vi "Diff Tree Items.vi"(10 "New Items":T1(array[cluster])=[{"Parent Tag"="", "Child Tag"="C:\\Users\\zwatx\\Developer\\LabView\\2026\\rebuilt-2687\\Robot Code\\Paths\\Choreo", "Left Cell Text"="Choreo", "Column Texts[]"=[], "Is File"=FALSE}, {"Parent Tag"="C:\\Users\\zwatx\\Developer\\LabView\\2026\\rebuilt-2687\\Robot Code\\Paths\\Choreo", "Child Tag"="C:\\Users\\zwatx\\Developer\\LabView\\2026\\rebuilt-2687\\Robot Code\\Paths\\Choreo\\Test", "Left Cell Text"="Test", "Column Texts[]"=[], "Is File"=FALSE}, {"Parent Tag"="", "Child Tag"="C:\\Users\\zwatx\\Developer\\LabView\\2026\\rebuilt-2687\\Robot Code\\Paths\\Hi", "Left Cell Text"="Hi", "Column Texts[]"=[], "Is File"=FALSE}], 11 "Old Items":T1(array[cluster])=[{"Parent Tag"="", "Child Tag"="C:\\Users\\zwatx\\Developer\\LabView\\2026\\rebuilt-2687\\Robot Code\\Paths\\Choreo", "Left Cell Text"="Choreo", "Column Texts[]"=[], "Is File"=FALSE}, {"Parent Tag"="C:\\Users\\zwatx\\Developer\\LabView\\2026\\rebuilt-2687\\Robot Code\\Paths\\Choreo", "Child Tag"="C:\\Users\\zwatx\\Developer\\LabView\\2026\\rebuilt-2687\\Robot Code\\Paths\\Choreo\\Test", "Left Cell Text"="Test", "Column Texts[]"=[], "Is File"=FALSE}, {"Parent Tag"="", "Child Tag"="C:\\Users\\zwatx\\Developer\\LabView\\2026\\rebuilt-2687\\Robot Code\\Paths\\Hi", "Left Cell Text"="Hi", "Column Texts[]"=[], "Is File"=FALSE}]) -> (1 "Removed Items":T1(array[cluster]), 2 "Changed Items":T1(array[cluster]), 3 "Added Items":T1(array[cluster]))   [LabVIEW 2025]
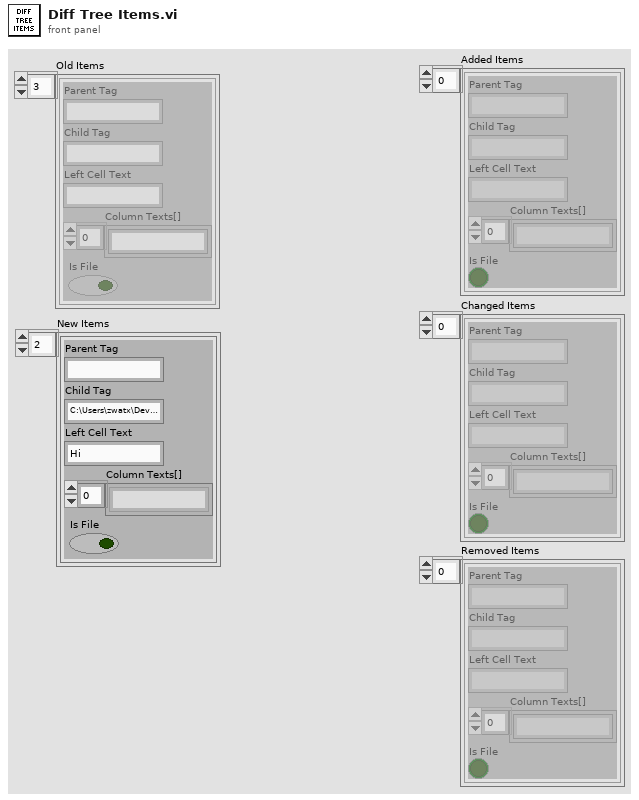
[diagram p1: front panel]
types:
  T1 = cluster{"Parent Tag":string, "Child Tag":string, "Left Cell Text":string, "Column Texts[]":string[], "Is File":bool}[]
  T2 = cluster{"Parent Tag":string, "Child Tag":string, "Left Cell Text":string, "Column Texts[]":string[], "Is File":bool}
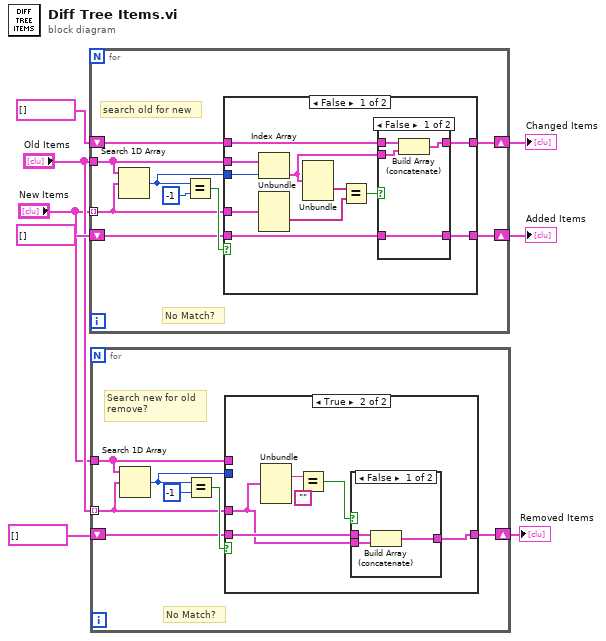
[diagram p0: block diagram]
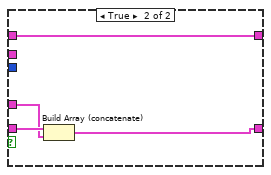
[diagram p5: hidden frame]
diagram:
  n1 = for {
    tunnel: "New Items" -> [w14] mode=indexing
    tunnel: "Old Items" -> [w12]
    shift-right: [w13] -> w7
    shift-left: T1 [] ("Old Items") -> [w15]
    shift-right: [w9] -> w5
    shift-left: T1 [] ("Old Items") -> [w10]
    # "search old for new"
    # "No Match?"
    n2 = Search 1D Array(1D array=w12, element=w14) -> (index of element=w11:i32)  [unwired: 1 in]
    n3 = Equal?(x=w11, y=-1) -> (x = y?=w16:bool)
    n4 = case shown="False" w16 {
      tunnel: w15 -> [w22 w38]
      tunnel: w14 -> [w26 w37]
      tunnel: [w21 w36] -> w13
      tunnel: w12 -> [w28 _]
      tunnel: w11 -> [w27 _]
      tunnel: w10 -> [w20 w35]
      tunnel: [w18 w35] -> w9
      frame False {
        n5 = Index Array(array=w28, index=w27) -> (element=w19:T2)
        n6 = Unbundle(w26) -> ("Column Texts[]"=w24:string[])  [unwired: 4 out]
        n7 = Unbundle(w19) -> ("Column Texts[]"=w25:string[])  [unwired: 4 out]
        n8 = Equal?(x=w25, y=w24) -> (x = y?=w23:bool)
        n9 = case shown="False" w23 {
          tunnel: w22 -> [w32 w34]
          tunnel: [w32 w34] -> w21
          tunnel: w20 -> [w31 w33]
          tunnel: w19 -> [w30 _]
          tunnel: [w29 w33] -> w18
          frame False {
            n10 = Build Array (concatenate)(w31, w30) -> (w29:T1)
          }
          frame True {
          }
        }
      }
      frame True {
        n11 = Build Array (concatenate)(w38, w37) -> (w36:T1)
      }
    }
  }
  "Added Items" <- w7
  "Changed Items" <- w5
  n12 = for {
    tunnel: "Old Items" -> [w42] mode=indexing
    tunnel: "New Items" -> [w39]
    shift-right: [w41] -> w1
    shift-left: T1 [] ("Old Items") -> [w43]
    # "Search new for old\nremove?"
    # "No Match?"
    n13 = Search 1D Array(1D array=w39, element=w42) -> (index of element=w40:i32)  [unwired: 1 in]
    n14 = Equal?(x=w40, y=-1) -> (x = y?=w44:bool)
    n15 = case shown="True" w44 {
      tunnel: w43 -> [w46 w52]
      tunnel: w42 -> [_ w50]
      tunnel: [w46 w51] -> w41
      tunnel: w39 -> [_ _]
      tunnel: w40 -> [_ _]
      frame False {
      }
      frame True {
        n16 = Unbundle(w50) -> ("Child Tag"=w49:string)  [unwired: 4 out]
        n17 = Equal?(x=w49, y="") -> (x = y?=w47:bool)
        n18 = case shown="False" w47 {
          tunnel: w52 -> [w55 w56]
          tunnel: [w54 w56] -> w51
          tunnel: w50 -> [w53 _]
          frame False {
            n19 = Build Array (concatenate)(w55, w53) -> (w54:T1)
          }
          frame True {
          }
        }
      }
    }
  }
  "Removed Items" <- w1
